vi "KH Control.vi"(11 "Channel Setting":T1(array[cluster])=[{"Channel"=1, "Gain"=4, "Shunt Resistor"=1, "Measure"=2}, {"Channel"=2, "Gain"=3, "Shunt Resistor"=5, "Measure"=1}, {"Channel"=3, "Gain"=3, "Shunt Resistor"=1, "Measure"=2}, {"Channel"=4, "Gain"=4, "Shunt Resistor"=1, "Measure"=2}, {"Channel"=5, "Gain"=4, "Shunt Resistor"=1, "Measure"=2}, {"Channel"=6, "Gain"=4, "Shunt Resistor"=5, "Measure"=1}, {"Channel"=7, "Gain"=3, "Shunt Resistor"=1, "Measure"=2}, {"Channel"=8, "Gain"=3, "Shunt Resistor"=5, "Measure"=1}] {"Measure" items=["Float", "Current(Diff)", "Voltage(SE+)"]; "Shunt Resistor" items=["Open"=1, "50 Ohms"=2, "500 Ohms"=3, "5k Ohms"=4, "50k Ohms"=5]; "Gain" items=["1x"=1, "10x"=2, "100x"=3, "1000x"=4]; "Channel" items=["Channel 1"=1, "Channel 2"=2, "Channel 3"=3, "Channel 4"=4, "Channel 5"=5, "Channel 6"=6, "Channel 7"=7, "Channel 8"=8]}) -> ()   [LabVIEW 2013]
panel:
  in  "VISA Refnum in":refnum<visa-resource-name>="COM3"
  # "Measure Current: Current, Shunt Resistor: 50kOhm\nMeasure Voltage: Voltage, Shunt Resistor: Open\nApplying Gate: Current, Shunt Resistor: 50kOhm\n                      Open all the unused gate"
  # "1. Create a copy of drivers under C:\\Krohn-Hite 7008\\Drivers if there is none. \n2. In device manager browse the driver for Krohn-Hite"
  # "Warning: repeated channels will cause false reading in the lock-in"
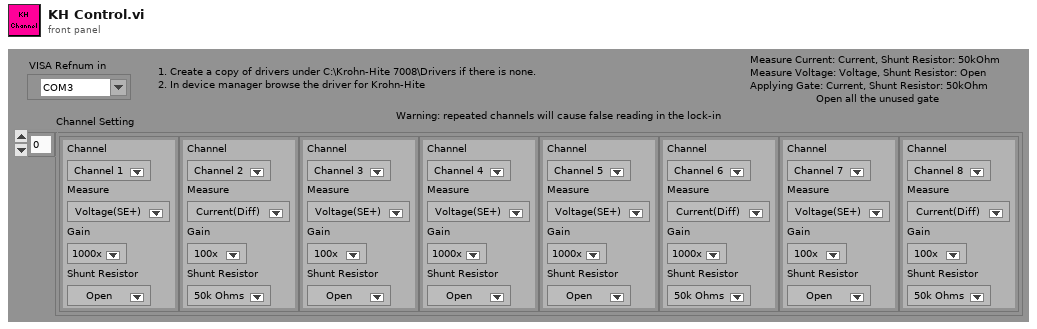
[diagram p1: front panel]
types:
  T1 = cluster{"Channel":u16, "Gain":u16, "Shunt Resistor":u16, "Measure":u16}[]
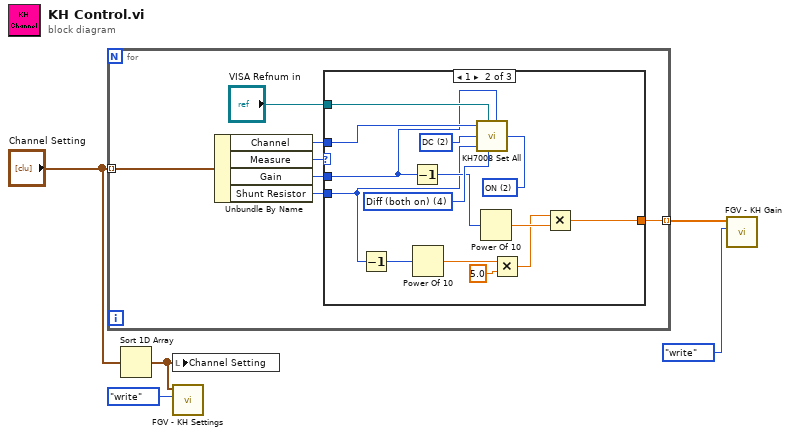
[diagram p0: block diagram]
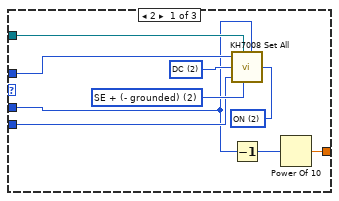
[diagram p2: hidden frame]
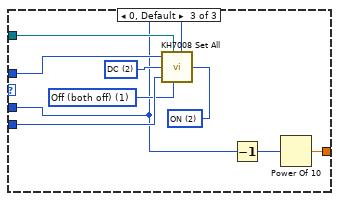
[diagram p3: hidden frame]
diagram:
  n1 = for {
    tunnel: "Channel Setting" -> [w8] mode=indexing
    tunnel: [w6] -> w2 mode=indexing
    n2 = Unbundle By Name(w8) -> ("Channel"=w11:u16, "Measure"=w7:u16, "Gain"=w10:u16, "Shunt Resistor"=w9:u16)
    n3 = case shown="1" w7 {
      tunnel: w11 -> [w18 w35 w44]
      tunnel: w10 -> [w14 w28 w37]
      tunnel: w9 -> [w17 w22 w42]
      tunnel: "VISA Refnum in" -> [w16 w31 w39]
      tunnel: [w13 w30 w36] -> w6
      frame 2 {
        w19 = u16 2 items=["Off (both off)"=1, "SE + (- grounded)"=2, "SE - (+ grounded)"=3, "Diff (both on)"=4] ("Input Coupling")
        w20 = u16 2 items=["OFF"=1, "ON"=2] ("Bandwidth Filter")
        w21 = u16 2 items=["AC"=1, "DC"=2] ("Coupling")
        n4 = call "KH7008 Set All.vi"("Channel"=w18, "VISA Refnum in"=w16, "Coupling"=w21, "Shunt Resistor"=w17, "Input Coupling"=w19, "Gain"=w14, "Bandwidth Filter"=w20) -> ()  [unwired: 2 in, 1 out]
        n5 = Decrement(x=w14) -> (x-1=w15:u16)
        n6 = Power Of 10(x=w15) -> (10^x=w13:dbl)
      }
      frame 1 {
        w32 = u16 2 items=["OFF"=1, "ON"=2] ("Bandwidth Filter")
        w33 = u16 4 items=["Off (both off)"=1, "SE + (- grounded)"=2, "SE - (+ grounded)"=3, "Diff (both on)"=4] ("Input Coupling")
        w34 = u16 2 items=["AC"=1, "DC"=2] ("Coupling")
        n7 = Decrement(x=w22) -> (x-1=w23:u16)
        n8 = Decrement(x=w28) -> (x-1=w29:u16)
        n9 = Power Of 10(x=w23) -> (10^x=w25:dbl)
        n10 = call "KH7008 Set All.vi"("Channel"=w35, "VISA Refnum in"=w31, "Coupling"=w34, "Shunt Resistor"=w22, "Input Coupling"=w33, "Gain"=w28, "Bandwidth Filter"=w32) -> ()  [unwired: 2 in, 1 out]
        n11 = Power Of 10(x=w29) -> (10^x=w27:dbl)
        n12 = Multiply(x=w25, y=5.0) -> (x*y=w24:dbl)
        n13 = Multiply(x=w24, y=w27) -> (x*y=w30:dbl)
      }
      frame 0, Default {
        w40 = u16 2 items=["OFF"=1, "ON"=2] ("Bandwidth Filter")
        w41 = u16 1 items=["Off (both off)"=1, "SE + (- grounded)"=2, "SE - (+ grounded)"=3, "Diff (both on)"=4] ("Input Coupling")
        w43 = u16 2 items=["AC"=1, "DC"=2] ("Coupling")
        n14 = call "KH7008 Set All.vi"("Channel"=w44, "VISA Refnum in"=w39, "Coupling"=w43, "Shunt Resistor"=w42, "Input Coupling"=w41, "Gain"=w37, "Bandwidth Filter"=w40) -> ()  [unwired: 2 in, 1 out]
        n15 = Decrement(x=w37) -> (x-1=w38:u16)
        n16 = Power Of 10(x=w38) -> (10^x=w36:dbl)
      }
    }
  }
  n17 = Sort 1D Array(array="Channel Setting") -> (sorted array=w4:T1)
  n18 = local write "Channel Setting"(w4) -> ()
  n19 = call "FGV - KH Settings.vi"("Function"=enum16{"write", "read"}."write", "Channel Setting"=w4) -> ()  [unwired: 4 in, 2 out]
  n20 = call "FGV - KH Gain.vi"("Function"=enum16{"write", "read"}."write", "Array"=w2) -> ()  [unwired: 4 in, 2 out]
